vi "_Raise Download Starting.vi"(4 "WebView2.lvlib:WebView2 Control.lvclass":refnum<class "WebView2 Control.lvclass">, 5 "Event Data":cluster{"sender":refnum<k24>, "e":refnum<k24>}, 6 "Control Ref":refnum<k24>, 7 "Event Common Data":T1) -> ()   [LabVIEW 2025, in "WebView2.lvlib" / "WebView2 Control.lvclass"]
uses:
  WebView2 Control.lvclass
  WebView2 Control.lvclass/WebView2 Control.ctl
  E:/Labview/LV 2023/PPL/PPL Builder/Libs/LV-WebView2/Source/Libs/Microsoft.Web.WebView2.Core.dll
  Libs/Microsoft.Web.WebView2.Core.dll
  WebView2 Event Filter Interface/WebView2 Event Filter Interface.lvclass
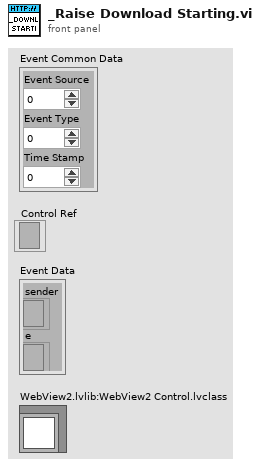
[diagram p1: front panel]
types:
  T1 = cluster{"Event Source":i32, "Event Type":u32, "Time Stamp":u32}
  T2 = cluster{"Cancel":bool, "Handled":bool, "ResultFilePath":string}
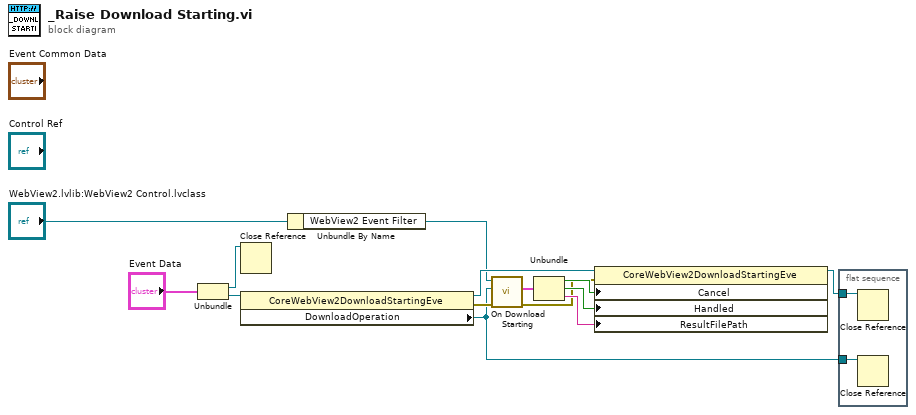
[diagram p0: block diagram]
diagram:
  n1 = Unbundle("Event Data") -> ("sender"=w13:refnum<k24>, "e"=w12:refnum<k24>)
  n2 = Close Reference(reference=w13) -> ()  [unwired: 1 in, 1 out]
  n3 = property class="CoreWebView2DownloadStartingEve"(reference=w12) -> (reference out=w10:refnum<k24>, error out=w8:errorcluster, "DownloadOperation"=w1:refnum<k24>)  [unwired: 1 in]
  n4 = Unbundle By Name("WebView2.lvlib:WebView2 Control.lvclass") -> ("WebView2 Event Filter"=w9:refnum<class "WebView2 Event Filter Interface.lvclass">)
  n5 = call-dynamic "On Download Starting.vi"("error in (no error)"=w8, "DownloadOperation"=w1, "WebView2 Event Filter Interface in"=w9) -> ("error out"=w2:errorcluster, "Response"=w7:T2)  [unwired: 7 in]
  n6 = Unbundle(w7) -> ("Cancel"=w6:bool, "Handled"=w5:bool, "ResultFilePath"=w4:string)
  n7 = property class="CoreWebView2DownloadStartingEve"(reference=w10, error in=w2, "Cancel"=w6, "Handled"=w5, "ResultFilePath"=w4) -> (reference out=w3:refnum<k24>)  [unwired: 1 out]
  n8 = flat-sequence {
    tunnel: w3 -> [w16]
    tunnel: w1 -> [w15]
    frame #0 {
      n9 = Close Reference(reference=w16) -> ()  [unwired: 1 in, 1 out]
      n10 = Close Reference(reference=w15) -> ()  [unwired: 1 in, 1 out]
    }
  }
